vi "FindButton.vi"() -> (0 "Handle":u64)   [LabVIEW 2014]
uses:
  user32.dll
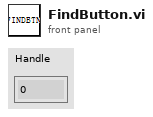
[diagram p1: front panel]
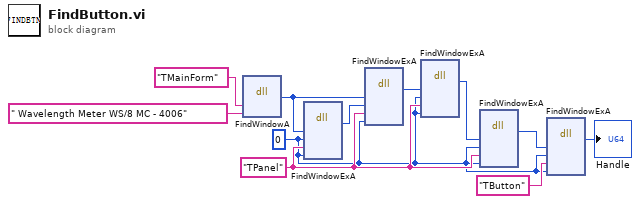
[diagram p0: block diagram]
diagram:
  w6 = "TPanel" ("arg1")
  w2 = u64 0 ("arg4")
  n1 = dll-call lib="user32.dll" fn="FindWindowA"("arg1"="TMainForm", "arg2"=" Wavelength Meter WS/8 MC - 4006") -> ("return type"=w9:u64)  [unwired: 5 in, 2 out]
  n2 = dll-call lib="user32.dll" fn="FindWindowExA"("arg3"=w9, "arg4"=w2, "arg1"=w6, "arg2"=w2) -> ("return type"=w8:u64)  [unwired: 7 in, 2 out]
  n3 = dll-call lib="user32.dll" fn="FindWindowExA"("arg3"=w9, "arg4"=w8, "arg1"=w6, "arg2"=w2) -> ("return type"=w5:u64)  [unwired: 7 in, 2 out]
  n4 = dll-call lib="user32.dll" fn="FindWindowExA"("arg3"=w5, "arg4"=w2, "arg1"=w6, "arg2"=w2) -> ("return type"=w7:u64)  [unwired: 7 in, 2 out]
  n5 = dll-call lib="user32.dll" fn="FindWindowExA"("arg3"=w7, "arg4"=w2, "arg1"=w6, "arg2"=w2) -> ("return type"=w4:u64)  [unwired: 7 in, 2 out]
  n6 = dll-call lib="user32.dll" fn="FindWindowExA"("arg3"=w4, "arg4"=w2, "arg1"="TButton", "arg2"=w2) -> ("return type"=→"Handle":u64)  [unwired: 7 in, 2 out]
